vi "solar.vi"() -> ()   [LabVIEW 2020]
uses:
  <vilib>/MakerHub/LINX/Public/Peripherals/PWM/PWM Set Duty Cycle 1 Chan.vi
  <vilib>/MakerHub/LINX/Public/Peripherals/Analog/Analog Read 1 Chan.vi
  <vilib>/MakerHub/LINX/Public/Peripherals/Analog/Analog Read N Chans.vi
  <vilib>/MakerHub/LINX/Private/Local IO/LinxAnalogRead.vi
  <vilib>/MakerHub/LINX/Public/Utilities/Check Channel.vi
  <vilib>/MakerHub/LINX/Public/Utilities/Open Serial.vi
  <vilib>/MakerHub/LINX/Private/Utilties/Generate Error.vi
  <vilib>/MakerHub/LINX/Public/Peripherals/PWM/PWM Set Duty Cycle N Chans.vi
  <vilib>/Utility/file.llb/Write Delimited Spreadsheet (DBL).vi
  <vilib>/MakerHub/LINX/LMH-LINX.lvlib
panel:
  out "XY Graph":cluster{"Y":dbl[], "Y":dbl[]}[](graph)
  out "?":dbl(graph)
  out "current photodiode mA":dbl(graph)
  out "Numeric":i32
  out "LED V":dbl
  out "Error Out 2":errorcluster
  out "Voltage":dbl
  in  "stop":bool
  out "Error Out":errorcluster
  in  "Slide":dbl(slide) scale=0.0..1.0
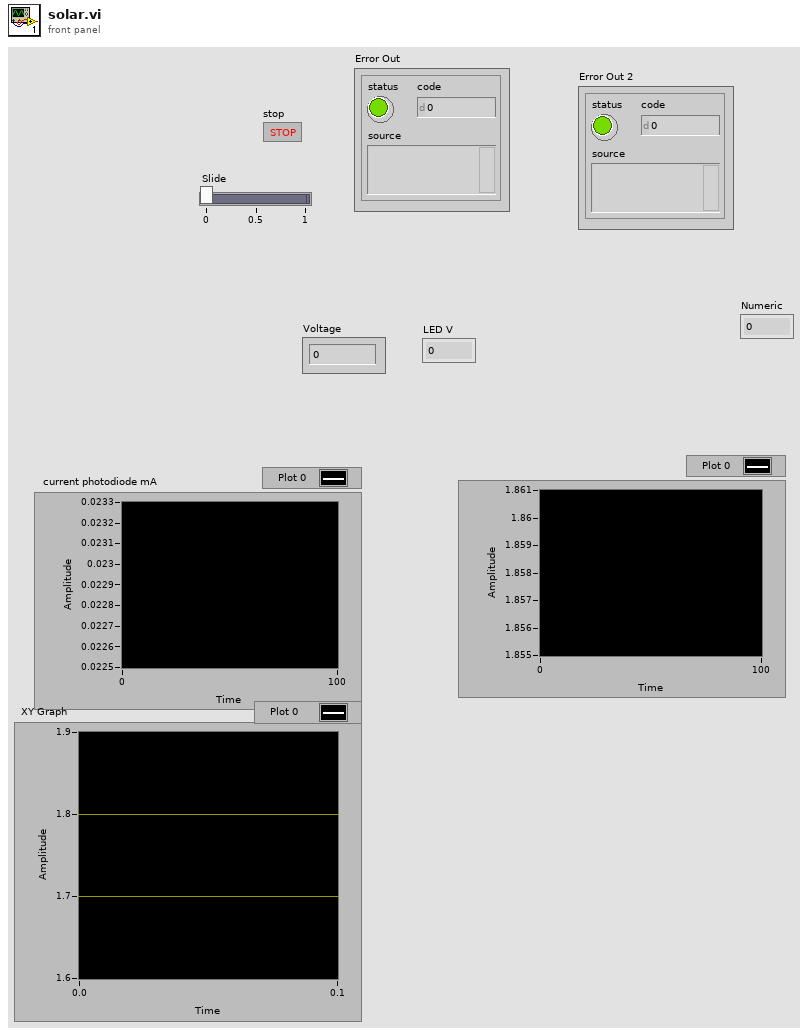
[diagram p1: front panel]
types:
  T1 = typedef "LMH-LINX.lvlib/LINX Ref.ctl" = cluster{"IO":T2, "Interface":T3, "LINX Device Config":T4}
  T2 = typedef "LMH-LINX.lvlib/Platform.ctl" = enum16{"Remote", "Local"}
  T3 = typedef "LMH-LINX.lvlib/Interface.ctl" = enum16{"Serial", "TCP"}
  T4 = typedef "LMH-LINX.lvlib/Device.lvlib/LINX Device Config.ctl" = cluster{"Interface":T3, "COM Port":refnum<visa-resource-name>, "TCP Configuration":T5, "Device Family":u8, "Device ID":u8, "Device Name":string, "TCP Ref":refnum<k5>, "Channels":T6}
  T5 = typedef "LMH-LINX.lvlib/Device.lvlib/TCP Config.ctl" = cluster{"IP Address":string, "Port":u16}
  T6 = typedef "LMH-LINX.lvlib/Channels.ctl" = cluster{"DI":u8[], "DO":u8[], "AI":u8[], "AO":u8[], "PWM":u8[], "QE":u8[], "UART":u8[], "I2C 2":u8[], "SPI":u8[], "CAN":u8[], "Servo":u8[], "AI Ref (V)":dbl, "AI Resolution (Bits)":u8, "AO Ref (V)":dbl, "AO Resolution (Bits)":u8}
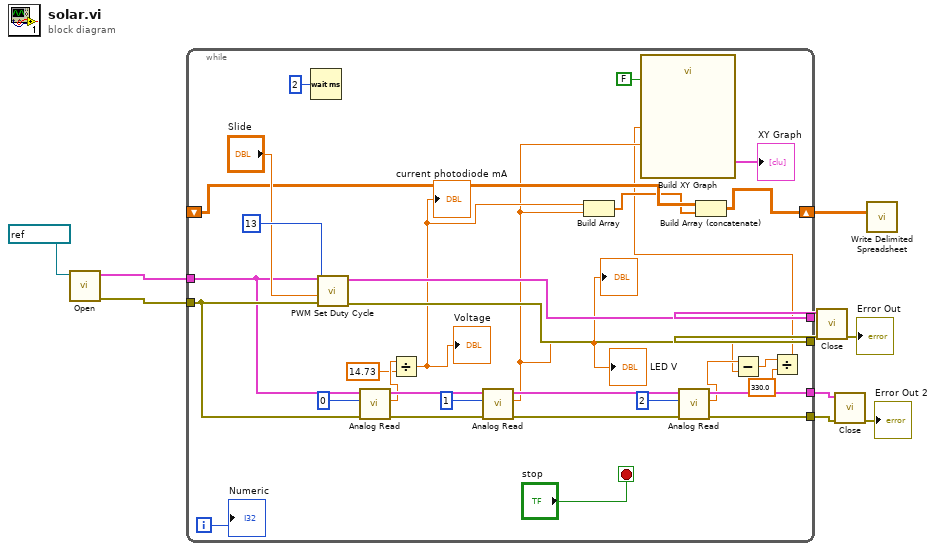
[diagram p0: block diagram]
diagram:
  n1 = call-poly <vilib>:"Open.vi"("Serial Port"=refnum<visa-resource-name> "COM4") -> ("Error Out"=w6:errorcluster, "LINX Resource"=w7:T1)  [unwired: 8 in, 1 out]
  n2 = while {
    tunnel: [w37] -> w10
    tunnel: [w41] -> w5
    tunnel: w7 -> [w34]
    tunnel: w6 -> [w35]
    tunnel: [w18] -> w2
    tunnel: [w17] -> w3
    shift-right: [w24] -> w1
    shift-left: _ -> [w26]
    i -> [w29]
    stop <- "stop" stop-if-true
    n3 = Wait (ms)(milliseconds to wait=u32 2) -> ()  [unwired: 1 out]
    n4 = call-poly <vilib>:"PWM Set Duty Cycle.vi"("Error In"=w35, "Duty Cycle (0-1)"="Slide", "PWM Channel"=u8 13, "LINX Resource"=w34) -> ("Error Out"=w41:errorcluster, "LINX Resource"=w37:T1)  [unwired: 6 in]
    n5 = call-poly <vilib>:"Analog Read.vi"("Error In"=w35, "Analog Channel"=u8 0, "LINX Resource"=w34) -> ("Error Out"=w32:errorcluster, "Voltage"=w28:dbl, "LINX Resource"=w33:T1)  [unwired: 5 in, 1 out]
    n6 = Divide(x=w28, y=14.73) -> (x/y=w22:dbl)
    "Voltage" <- w22
    "current photodiode mA" <- w22
    n7 = call-poly <vilib>:"Analog Read.vi"("Error In"=w32, "Analog Channel"=u8 1, "LINX Resource"=w33) -> ("Error Out"=w19:errorcluster, "Voltage"=w14:dbl, "LINX Resource"=w20:T1)  [unwired: 5 in, 1 out]
    "LED V" <- w14
    "?" <- w14
    n8 = Build Array(w22, w14) -> (w25:dbl[])
    n9 = call-poly <vilib>:"Analog Read.vi"("Error In"=w19, "Analog Channel"=u8 2, "LINX Resource"=w20) -> ("Error Out"=w18:errorcluster, "Voltage"=w15:dbl, "LINX Resource"=w17:T1)  [unwired: 5 in, 1 out]
    n10 = Build Array (concatenate)(w26, w25) -> (w24:dbl[][])
    n11 = Subtract(x=w15, y=w14) -> (x-y=w13:dbl)
    n12 = Divide(x=w13, y=330.0) -> (x/y=w11:dbl)
    n13 = call "Build XY Graph"("Reset"=FALSE, "Y Input"=w14, "X Input"=w11) -> ("XY Graph"=→"XY Graph":cluster{"X":dbl[], "Y":dbl[]}[])  [unwired: 7 in, 1 out]
    "Numeric" <- w29
  }
  n14 = call <vilib>:"Close.vi"("Error In"=w5, "LINX Resource"=w10) -> ("Error Out"=→"Error Out":errorcluster)  [unwired: 9 in]
  n15 = call <vilib>:"Close.vi"("Error In"=w2, "LINX Resource"=w3) -> ("Error Out"=→"Error Out 2":errorcluster)  [unwired: 9 in]
  n16 = call-poly <vilib>:"Write Delimited Spreadsheet.vi"("2D data"=w1) -> ()  [unwired: 13 in, 2 out]
